vi "_f_bronkhorstRead.vi"(8 "error in (no error)":errorcluster) -> (0 "error out":errorcluster, 1 "Dispositivos":T1=[["3", "NO", "M0000013", "Air", "1", "ln/mn", "0", "0"], ["4", "NO", "M0000014", "Air", "1", "ln/mn", "0", "0"], ["5", "NO", "M0000015", "Air", "1", "ln/mn", "0", "0"], ["6", "NO", "M0000016", "Air", "1", "ln/mn", "0", "0"], ["7", "NO", "M0000017", "Air", "1", "ln/mn", "0", "0"], ["8", "NO", "M0000018", "Air", "1", "ln/mn", "0", "0"], ["9", "NO", "M0000019", "Air", "1", "ln/mn", "0", "0"], ["10", "NO", "M0000020", "Air", "1", "ln/mn", "0", "0"], ["11", "NO", "M0000021", "Air", "1", "ln/mn", "0", "0"]] caption="MassFlowControllers")   [LabVIEW 2013]
uses:
  _f_TablaBronkhorst.ctl
  _f_BronkhorstModuleControl.ctl
  P2022 TB INCAR GLOBALES.vi
panel:
  out "Enable(T)":bool=TRUE
  out "VISA Bronkhorst":refnum<visa-resource-name>
  in  "Delay Time (s)":dbl=0.1
  out "Num. of nodes":u32=6
  # "Reading setpoint and flow"
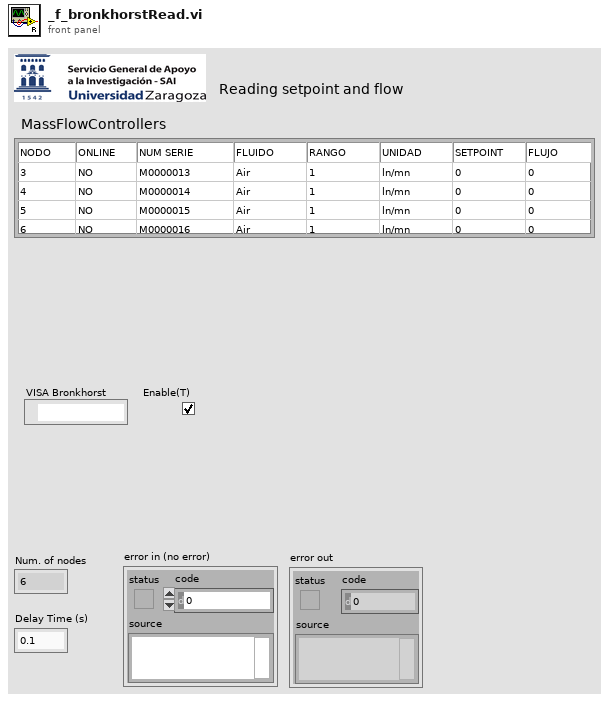
[diagram p1: front panel]
types:
  T1 = typedef "_f_TablaBronkhorst.ctl" = string[][]
  T2 = typedef "P2018 Bronkhorst Control.ctl" = cluster{"Dispositivos":T3, "NuevosSP":string[][], "Nodes":u32, "Delay(s)":dbl}
  T3 = typedef "_s_TablaBronkhorst.ctl" = string[][]
  T4 = typedef "P2018 Com Control.ctl" = cluster{"Flujo_1":refnum<visa-resource-name>, "Brk1":bool, "Flujo_2":refnum<visa-resource-name>, "Brk2":bool, "Flujo_3":refnum<visa-resource-name>, "Brk3":bool, "Flujo_4":refnum<visa-resource-name>, "Brk4":bool, "Eurothe":refnum<visa-resource-name>, "Eurot":bool, "Balanza":refnum<visa-resource-name>, "Bal":bool, "eValPos":refnum<visa-resource-name>, "eVal":bool, "flowbus":refnum<visa-resource-name>, "fb":bool}
  T5 = typedef "_f_BronkhorstModuleControl.ctl" = enum16{"RcharSerialNum", "RcharIdnString", "WuintFluidNum", "RuintFluidNum", "RcharFluidName", "RuintSensorType", "RfloatCap0", "RfloatCap100", "RcharCapUnitStr", "W%Setpoint", "R%Setpoint", "R%Measure", "WfloatSetpoint", "RfloatSetpoint", "RfloatMeasure ", "RfloatDensity", "WuintControlMode", "WcharRESET", "RfloatCounter", "RcharCounterUnit", "WfloatCounterLimit", "RfloatCounterLimit", "WcharCounterMode", "RcharCounterMode", "WcharCounterSPMode", "RcharCounterSPMode", "WcharCounterNewSP", "RcharCounterNewSP"}
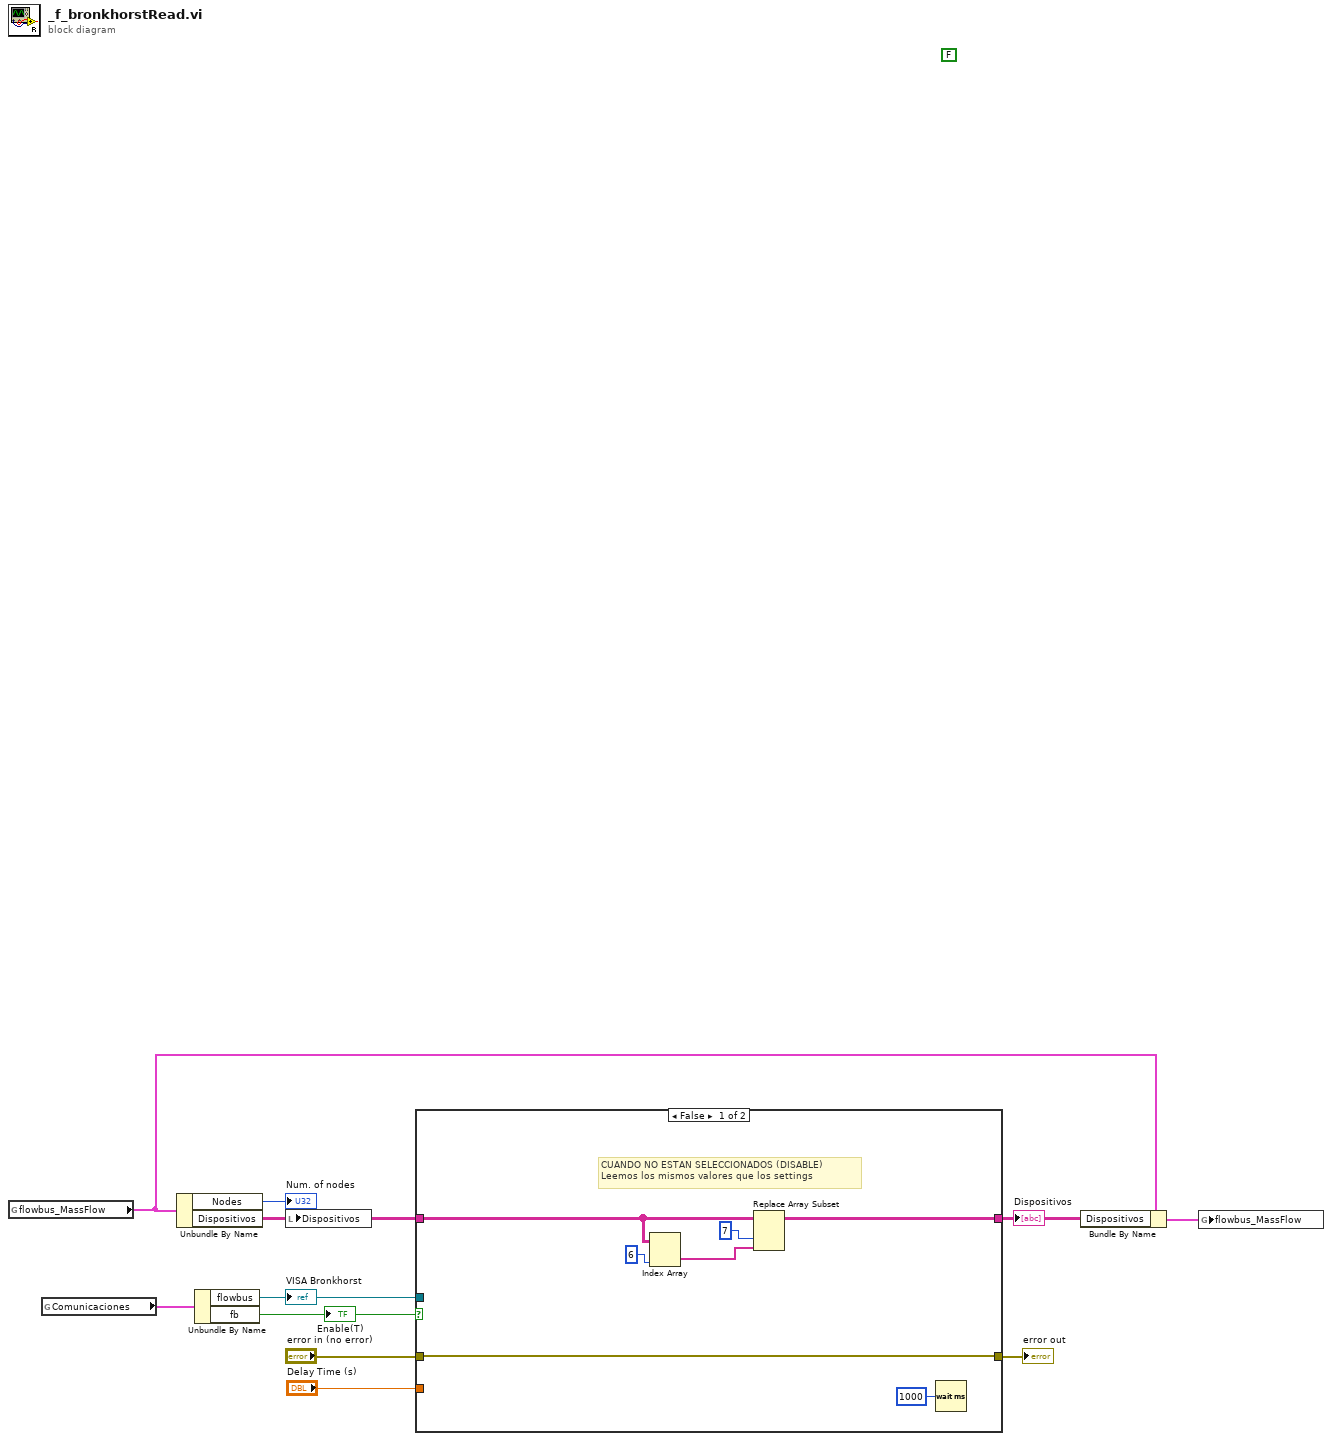
[diagram p0: block diagram]
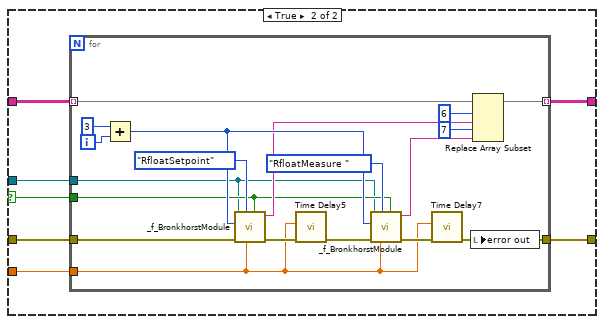
[diagram p2: hidden frame]
diagram:
  (unwired) FALSE
  n1 = global read "P2022 TB INCAR GLOBALES.vi" "flowbus_MassFlow"() -> (w1:T2)
  n2 = global read "P2022 TB INCAR GLOBALES.vi" "Comunicaciones"() -> (w11:T4)
  n3 = Unbundle By Name(w1) -> ("Nodes"=→"Num. of nodes":u32, "Dispositivos"=w4:T3)
  n4 = Unbundle By Name(w11) -> ("flowbus"=w9:refnum<visa-resource-name>, "fb"=w10:bool)
  "Enable(T)" <- w10
  "VISA Bronkhorst" <- w9
  n5 = local write "Dispositivos"(w4) -> ()
  n6 = case shown="False" w10 {
    selector: w10 -> [_ w20]
    tunnel: w9 -> [_ w19]
    tunnel: [w14 w23] -> w7
    tunnel: [w17 w25] -> w6
    tunnel: w4 -> [w15 w24]
    tunnel: "error in (no error)" -> [w17 w22]
    tunnel: "Delay Time (s)" -> [_ w21]
    frame False {
      # "CUANDO NO ESTAN SELECCIONADOS (DISABLE)\nLeemos los mismos valores que los settings"
      n7 = Index Array(array=w15, index (col)=6 ("index")) -> (element=w16:string[])  [unwired: 1 in]
      n8 = Replace Array Subset(array=w15, new element=w16, index (col)=7 ("index")) -> (w14:T3)  [unwired: 1 in]
      n9 = Wait (ms)(milliseconds to wait=u32 1000) -> ()  [unwired: 1 out]
    }
    frame True {
      n10 = for {
        tunnel: w22 -> [w34]
        tunnel: [w35] -> w25
        tunnel: w21 -> [w36]
        tunnel: w24 -> [w33] mode=indexing
        tunnel: [w30] -> w23 mode=indexing
        tunnel: w20 -> [w27]
        tunnel: w19 -> [w26]
        i -> [w43]
        n11 = Add(x=3, y=w43) -> (x+y=w37:i32)
        n12 = call "_f_BronkhorstModule.vi"("Enable(T)"=w27, "Delay"=w36, "Command"=_f_BronkhorstModuleControl."RfloatSetpoint", "error in (no error)"=w34, "Nodo"=w37, "VISA resource name"=w26) -> ("error out"=w41:errorcluster, "Value"=w29:string)  [unwired: 2 in, 2 out]
        n13 = call "Time Delay5"("error in (no error)"=w41, "Delay Time (s)"=w36) -> ("error out"=w38:errorcluster)  [unwired: 9 in]
        n14 = call "_f_BronkhorstModule.vi"("Enable(T)"=w27, "Delay"=w36, "Command"=_f_BronkhorstModuleControl."RfloatMeasure ", "error in (no error)"=w38, "Nodo"=w37, "VISA resource name"=w26) -> ("error out"=w39:errorcluster, "Value"=w28:string)  [unwired: 2 in, 2 out]
        n15 = call "Time Delay7"("error in (no error)"=w39, "Delay Time (s)"=w36) -> ("error out"=w35:errorcluster)  [unwired: 9 in]
        n16 = local write "error out"(w35) -> ()
        n17 = Replace Array Subset(array=w33, new element #1=w29, index #1=6 ("index"), new element #2=w28, index #2=7 ("index")) -> (w30:string[])
      }
    }
  }
  "error out" <- w6
  "Dispositivos" <- w7
  n18 = Bundle By Name(cluster=w1, "Dispositivos"=w7) -> (w8:T2)
  n19 = global write "P2022 TB INCAR GLOBALES.vi" "flowbus_MassFlow"(w8) -> ()
